vi "Create Class ObjectData DVR.vi"(8 "error in (no error)":errorcluster, 11 "DbgTimers in":refnum<class "DbgTimers.lvclass">) -> (0 "error out":errorcluster, 3 "DbgTimers out":refnum<class "DbgTimers.lvclass">)   [LabVIEW 2017, in "DbgTimers.lvclass"]
doc: "Developed by Kevin Thompson\nkevin@thompsonengineering.net\n\nCopyright 2018-2020\nThompson Engineering, LLC"
uses:
  DbgTimers.lvclass
  DataTypes/ObjData--cluster.ctl
  DataTypes/Settings--cluster.ctl
  DataTypes/Read Data--cluster.ctl
  DataTypes/Timers--cluster.ctl
  DataTypes/Millisecond Tick Timer--cluster.ctl
  DbgTimers.lvclass/DbgTimers.ctl
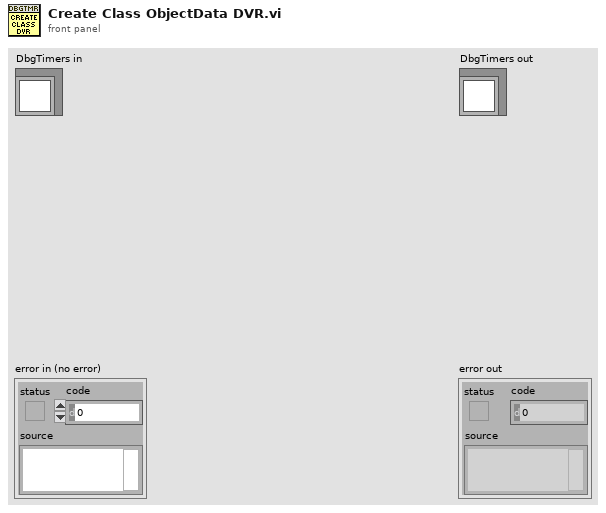
[diagram p1: front panel]
types:
  T1 = typedef "DbgTimers.lvclass/ObjData--cluster.ctl" = cluster{"Settings":T2, "ReadData-placeholder":T3, "Timers":T4, "Enable msTick Logging":bool, "LogFile_msTickTimer":path}
  T2 = typedef "DbgTimers.lvclass/Settings--cluster.ctl" = cluster{"Simulation":bool, "DbgTimer LogFolder":path}
  T3 = typedef "DbgTimers.lvclass/Read Data--cluster.ctl" = cluster{"Data":dbl}
  T4 = typedef "DbgTimers.lvclass/Timers--cluster.ctl" = cluster{"ms tick timers":T5[]}
  T5 = typedef "DbgTimers.lvclass/Millisecond Tick Timer--cluster.ctl" = cluster{"startTick":u32, "currentTick":u32, "elapsedTicks":u32, "totalElapsedTicks":u32}
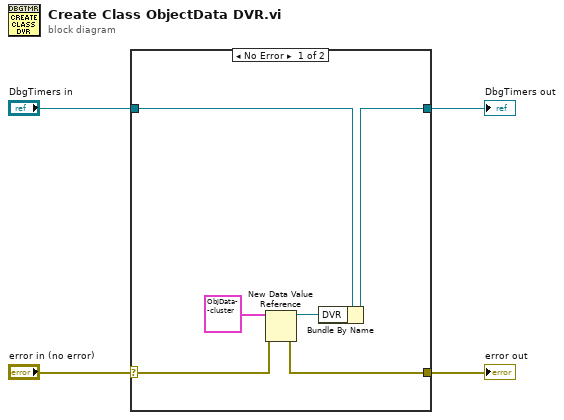
[diagram p0: block diagram]
diagram:
  n1 = case shown="No Error" "error in (no error)" {
    selector: "error in (no error)" -> [w9 w12]
    tunnel: [w8 w12] -> w3
    tunnel: [w6 w11] -> w1
    tunnel: "DbgTimers in" -> [w7 w11]
    frame No Error {
      n2 = New Data Value Reference(data value=T1 {"Settings"={"Simulation"=FALSE, "DbgTimer LogFolder"=path ""}, "ReadData-placeholder"={"Data"=0.0}, "Timers"={"ms tick timers"=[]}, "Enable msTick Logging"=FALSE, "LogFile_msTickTimer"=path ""} ("ObjData"), error in=w9) -> (data value reference=w10:refnum<data-value>, error out=w8:errorcluster)
      n3 = Bundle By Name(cluster=w7, "DVR"=w10) -> (w6:refnum<class "DbgTimers.lvclass">)
    }
    frame Error {
    }
  }
  "error out" <- w3
  "DbgTimers out" <- w1
